vi "Clear All.vi"(8 "error in":errorcluster, 11 "34980A in":refnum<class "34980A.lvclass">) -> (0 "error out":errorcluster, 3 "34980A out":refnum<class "34980A.lvclass">)   [LabVIEW 2019, in "34980A.lvlib" / "34980A.lvclass"]
uses:
  Library/34980A.lvclass
  builds/Instruments/MLTFNC.lvlibp/Library/MLTFNC.lvclass
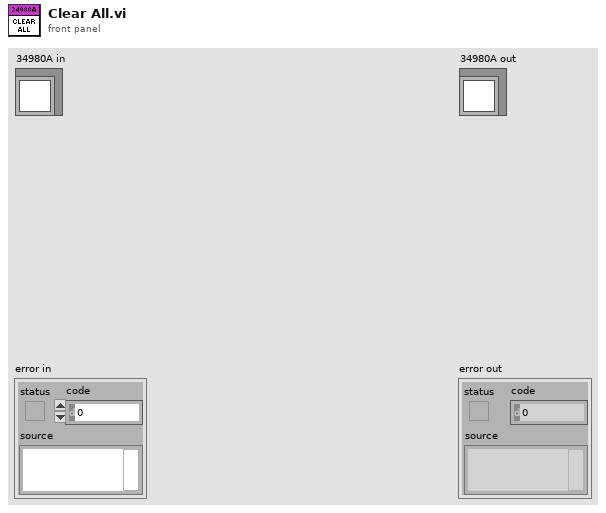
[diagram p1: front panel]
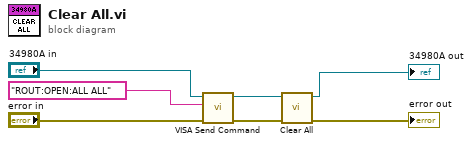
[diagram p0: block diagram]
diagram:
  n1 = call "VISA Send Command.vi"("error in"="error in", "Command"="ROUT:OPEN:ALL ALL", "34980A in"="34980A in") -> ("error out"=w3:errorcluster, "34980A out"=w2:refnum<class "34980A.lvclass">)  [unwired: 7 in]
  n2 = call-parent "Clear All.vi"("error in"=w3, "MLTFNC in"=w2) -> ("error out"=→"error out":errorcluster, "MLTFNC out"=→"34980A out":refnum<class "34980A.lvclass">)  [unwired: 8 in]
